vi "Smart IO Initialize Mode.vi"(8 "error in (no error)":errorcluster, 10 "mode":T1, 11 "deviceIndex":i32=-1) -> (0 "error out":errorcluster)   [LabVIEW 2026, in "MrcLib.lvlib"]
doc: "Configures the indicated device channel for a specific mode of I/O operation."
uses:
  MrcLib.lvlib
  Types/MRC Smart IO Mode.ctl
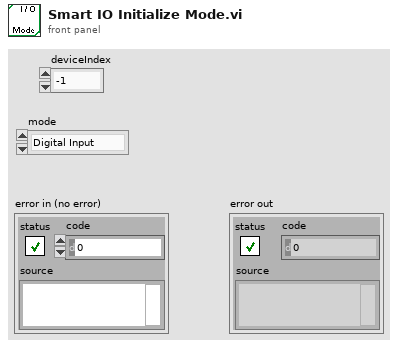
[diagram p1: front panel]
types:
  T1 = typedef "MRC Smart IO Mode.ctl" = i32
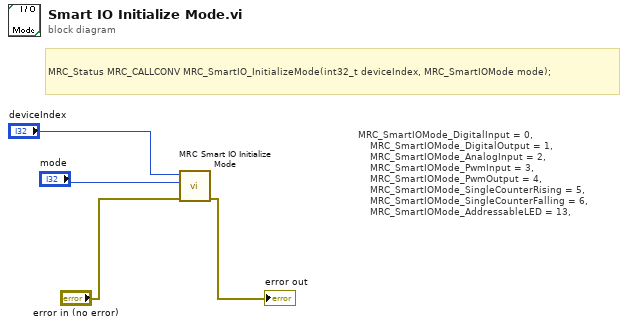
[diagram p0: block diagram]
diagram:
  # "MRC_SmartIOMode_DigitalInput = 0,\n    MRC_SmartIOMode_DigitalOutput = 1,\n    MRC_SmartIOMode_AnalogInput = 2,\n    MRC_SmartIOMode_PwmInput = 3,\n    MRC_SmartIOMode_PwmOutput = 4,\n    MRC_SmartIOMode_SingleCounterRising = 5,\n    MRC_SmartIOMode_SingleCounterFalling = 6,\n    MRC_SmartIOMode_AddressableLED = 13,"
  # "MRC_Status MRC_CALLCONV MRC_SmartIO_InitializeMode(int32_t deviceIndex, MRC_SmartIOMode mode);"
  n1 = call "MRC Smart IO Initialize Mode.vi"("error in (no error)"="error in (no error)", "mode"="mode", "deviceIndex"="deviceIndex") -> ("error out"=→"error out":errorcluster)  [unwired: 8 in]
